vi "CALC_TRAN_TIME_STIM.vi"(0 "VISA IN":refnum<visa-resource-name>, 1 "Stimulus":string, 5 "error in":errorcluster, 7 "Channel":i32) -> (14 "VISA Out":refnum<visa-resource-name>, 19 "error out":errorcluster)   [LabVIEW 2018, in "PNA-X.lvlib"]
doc: "CALCulate<cnum>:TRANsform:TIME:STIMulus <char> \n(Read-Write) Sets the type of simulated stimulus that will be incident on the DUT. \nSee Critical Note \nParameters \n<cnum> Channel number of the measurement. There must be a selected measurement \non that channel. If unspecified, <cnum> is set to 1. \n<char> Choose from: \nSTEP - simulates a step DUT stimulus \nIMPulse - simulates a pulse DUT stimulus \nSTEP can ONLY be used when CALC:TRAN:TIME:TYPE is set to LPASs \n(Lowpass). (STEP cannot be used with TYPE = BPASs.) \n:STIM STEP will set :TYPE to LPASs \n:TYPE BPASs will set :STIM to IMPulse \nExamples CALC:TRAN:TIME:STIM STEP \ncalculate2:transform:time:stimulus impulse \nQuery Syntax CALCulate<cnum>:TRANsform:TIME:STIMulus? \nReturn Type Character \n1573\n\nDefault IMPulse"
uses:
  PNA-X.lvlib
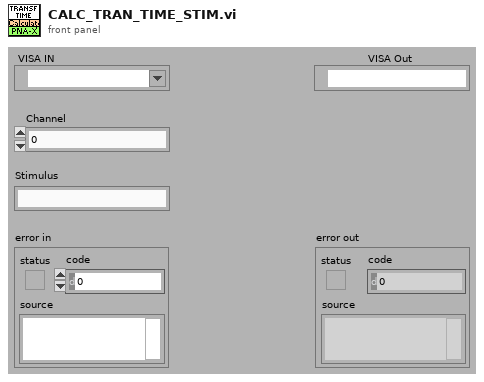
[diagram p1: front panel]
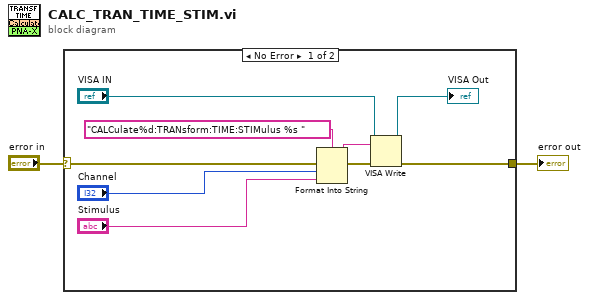
[diagram p0: block diagram]
diagram:
  n1 = case shown="No Error" "error in" {
    selector: "error in" -> [w11 w12]
    tunnel: [w6 w12] -> w1
    frame No Error {
      n2 = Format Into String(format string="CALCulate%d:TRANsform:TIME:STIMulus %s " ("Cmdline"), error in=w11, "Channel", "Stimulus") -> (resulting string=w9:string, error out=w10:errorcluster)  [unwired: 1 in]
      n3 = VISA Write(VISA resource name="VISA IN", write buffer=w9, error in (no error)=w10) -> (VISA resource name out=→"VISA Out":refnum<visa-resource-name>, error out=w6:errorcluster)  [unwired: 1 out]
    }
    frame Error {
    }
  }
  "error out" <- w1
